vi "cycleFreqCell.vi"(0 "emptyCorrArr":dbl[][](array[numeric]), 1 "emptyVarCorArr":dbl[](array[numeric]), 2 "signalArrayCDB":cdb[](array[numeric]), 3 "iFreq":dbl, 4 "Freq min":dbl, 5 "Freq cell":dbl, 6 "sampTime Array":dbl[](array[numeric]), 7 "fftCodeRefConj":cdb[](array[numeric]), 8 "numCellFreq":i32) -> (19 "Waveform Graph":dbl[](graph), 20 "corrArr":dbl[][](array[numeric]), 24 "ArrVarCor":dbl[](array[numeric]))   [LabVIEW 2020]
uses:
  <vilib>/Analysis/2dsp.llb/Complex FFT.vi
  <vilib>/Analysis/2dsp.llb/Inverse Complex FFT.vi
  <vilib>/Analysis/NI_AALPro.lvlib
  <vilib>/Analysis/NI_AALBase.lvlib
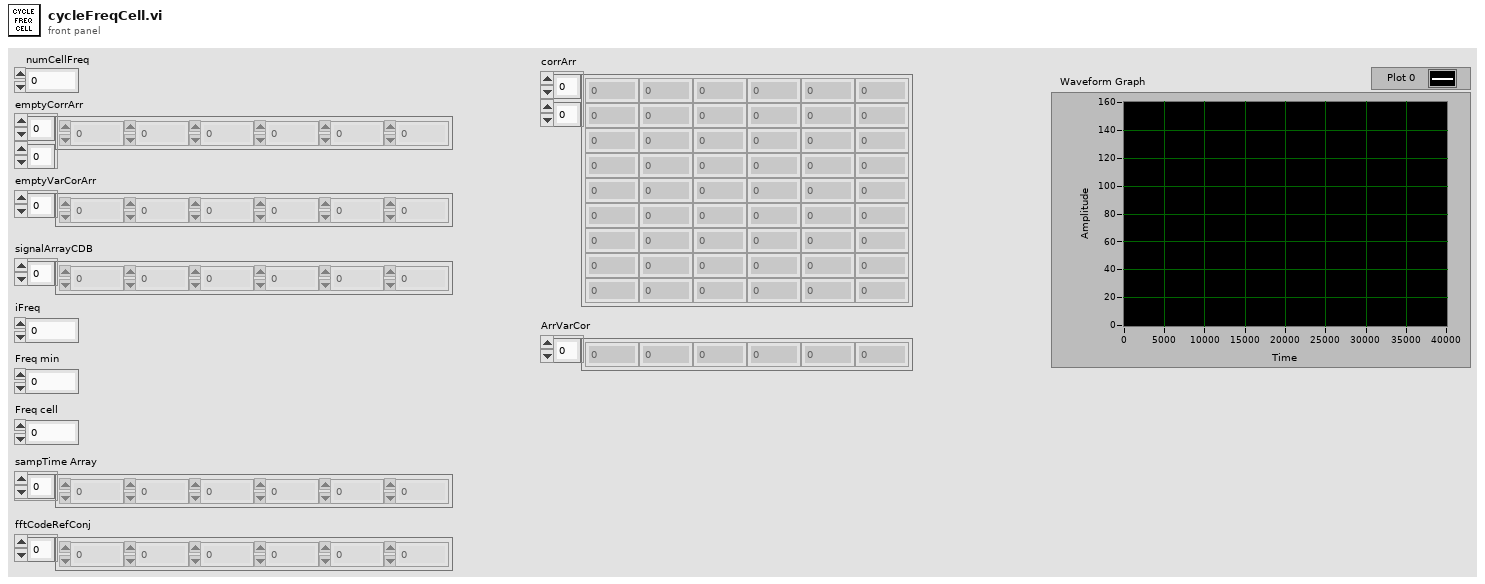
[diagram p1: front panel]
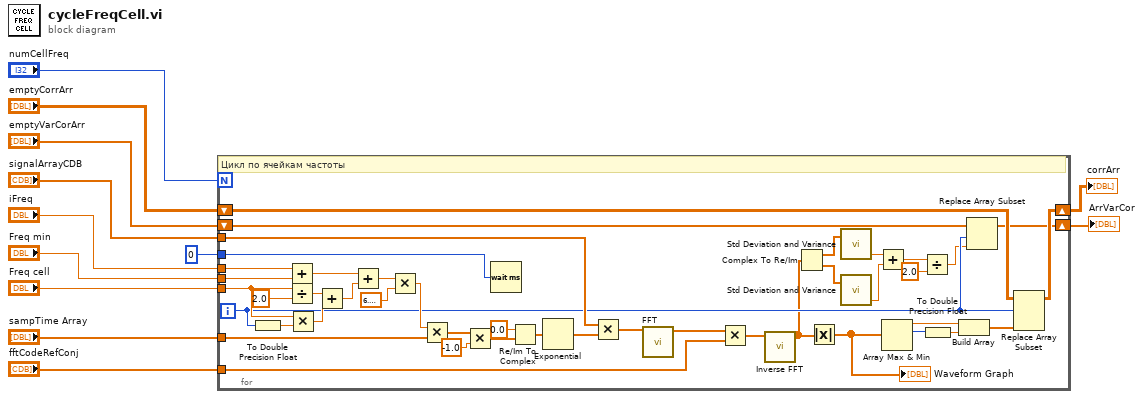
[diagram p0: block diagram]
diagram:
  n1 = for {
    N: "numCellFreq" -> [_]
    shift-right: [w28] -> w3
    shift-left: "emptyCorrArr" -> [w30]
    tunnel: "Freq min" -> [w55]
    tunnel: "iFreq" -> [w54]
    tunnel: "Freq cell" -> [w50]
    tunnel: "sampTime Array" -> [w44]
    tunnel: "signalArrayCDB" -> [w37]
    shift-right: [w25] -> w2
    shift-left: "emptyVarCorArr" -> [w27]
    tunnel: "fftCodeRefConj" -> [w23]
    tunnel: u32 0 ("milliseconds to wait") -> [w13]
    i -> [w26]
    # "Цикл по ячейкам частоты"
    n2 = To Double Precision Float(number=w26) -> (double precision float=w51:dbl)
    n3 = Add(x=w54, y=w55) -> (x+y=w48:dbl)
    n4 = Divide(x=w50, y=2.0) -> (x/y=w52:dbl)
    n5 = Multiply(x=w50, y=w51) -> (x*y=w49:dbl)
    n6 = Add(x=w52, y=w49) -> (x+y=w47:dbl)
    n7 = Add(x=w48, y=w47) -> (x+y=w46:dbl)
    n8 = Multiply(x=w46, y=6.283185307179586) -> (x*y=w43:dbl)
    n9 = Multiply(x=w43, y=w44) -> (x*y=w42:dbl[])
    n10 = Multiply(x=w42, y=-1.0) -> (x*y=w40:dbl[])
    n11 = Wait (ms)(milliseconds to wait=w13) -> ()  [unwired: 1 out]
    n12 = Re/Im To Complex(1:w40, 2:0.0) -> (0:w39:cdb[])
    n13 = Exponential(1:w39) -> (0:w38:cdb[])
    n14 = Multiply(x=w37, y=w38) -> (x*y=w36:cdb[])
    n15 = call-poly <vilib>:"FFT.vi"("X"=w36) -> ("FFT {X}"=w35:cdb[])  [unwired: 9 in, 1 out]
    n16 = Multiply(x=w35, y=w23) -> (x*y=w34:cdb[])
    n17 = call-poly <vilib>:"Inverse FFT.vi"("FFT {X}"=w34) -> ("X"=w20:cdb[])  [unwired: 9 in, 1 out]
    n18 = Complex To Re/Im(x + iy=w20) -> (x=w19:dbl[], y=w18:dbl[])
    n19 = Absolute Value(x=w20) -> (abs(x)=w14:dbl[])
    "Waveform Graph" <- w14
    n20 = call <vilib>:"Std Deviation and Variance.vi"("X"=w19) -> ("variance"=w17:dbl)  [unwired: 1 in, 2 out]
    n21 = call <vilib>:"Std Deviation and Variance.vi"("X"=w18) -> ("variance"=w16:dbl)  [unwired: 1 in, 2 out]
    n22 = Add(x=w17, y=w16) -> (x+y=w15:dbl)
    n23 = Array Max & Min(array=w14) -> (max value=w33:dbl, max index (indices)=w31:i32)  [unwired: 2 out]
    n24 = Divide(x=w15, y=2.0) -> (x/y=w21:dbl)
    n25 = To Double Precision Float(number=w31) -> (double precision float=w32:dbl)
    n26 = Build Array(w33, w32) -> (w29:dbl[])
    n27 = Replace Array Subset(array=w27, new element=w21, index=w26) -> (w25:dbl[])
    n28 = Replace Array Subset(array=w30, new element=w29, index (row)=w26) -> (w28:dbl[][])  [unwired: 1 in]
  }
  "corrArr" <- w3
  "ArrVarCor" <- w2
